vi "drawVessel.vi"(2 "alpha":dbl[](array[numeric]), 3 "u":dbl[](array[numeric])) -> (1 "?":picture)   [LabVIEW 2014]
uses:
  <vilib>/imath/engines/lvmath2/RunTimeEngine/NodeEndStatement/NIMS_NodeEndStatement_Output.vi
  <instcachedir>/0/NIMS_NodeEndStatement_Output_53EC0D466D134D7ABD903AC30B43404B.lvgen/NIMS_NodeEndStatement_Output_53EC0D466D134D7ABD903AC30B43404B_001.vi
  <vilib>/imath/engines/lvmath2/RunTimeEngine/ErrorHandling/NIMS_Finalize Error.vi
panel:
  out "?":picture
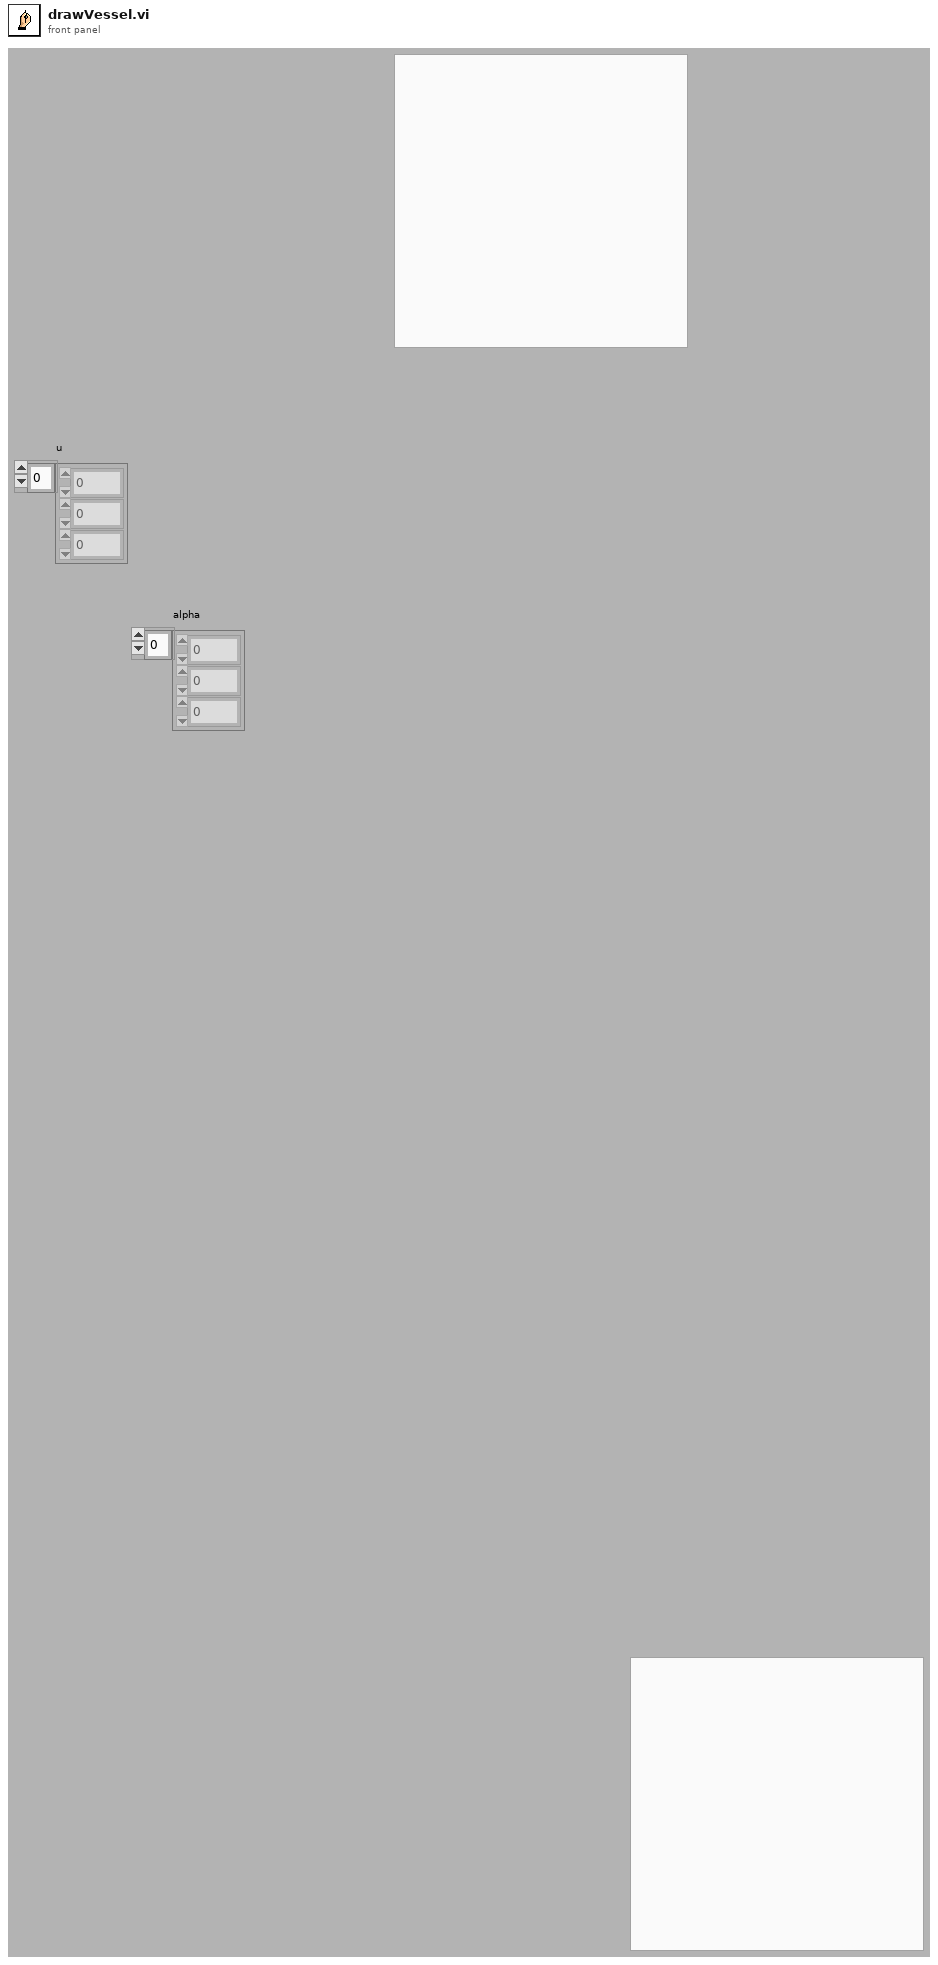
[diagram p1: front panel]
types:
  T1 = cluster{"Width":u16, "Style":enum32{"Solid", "Dash", "Dot", "DashDot", "DashDotDot"}}
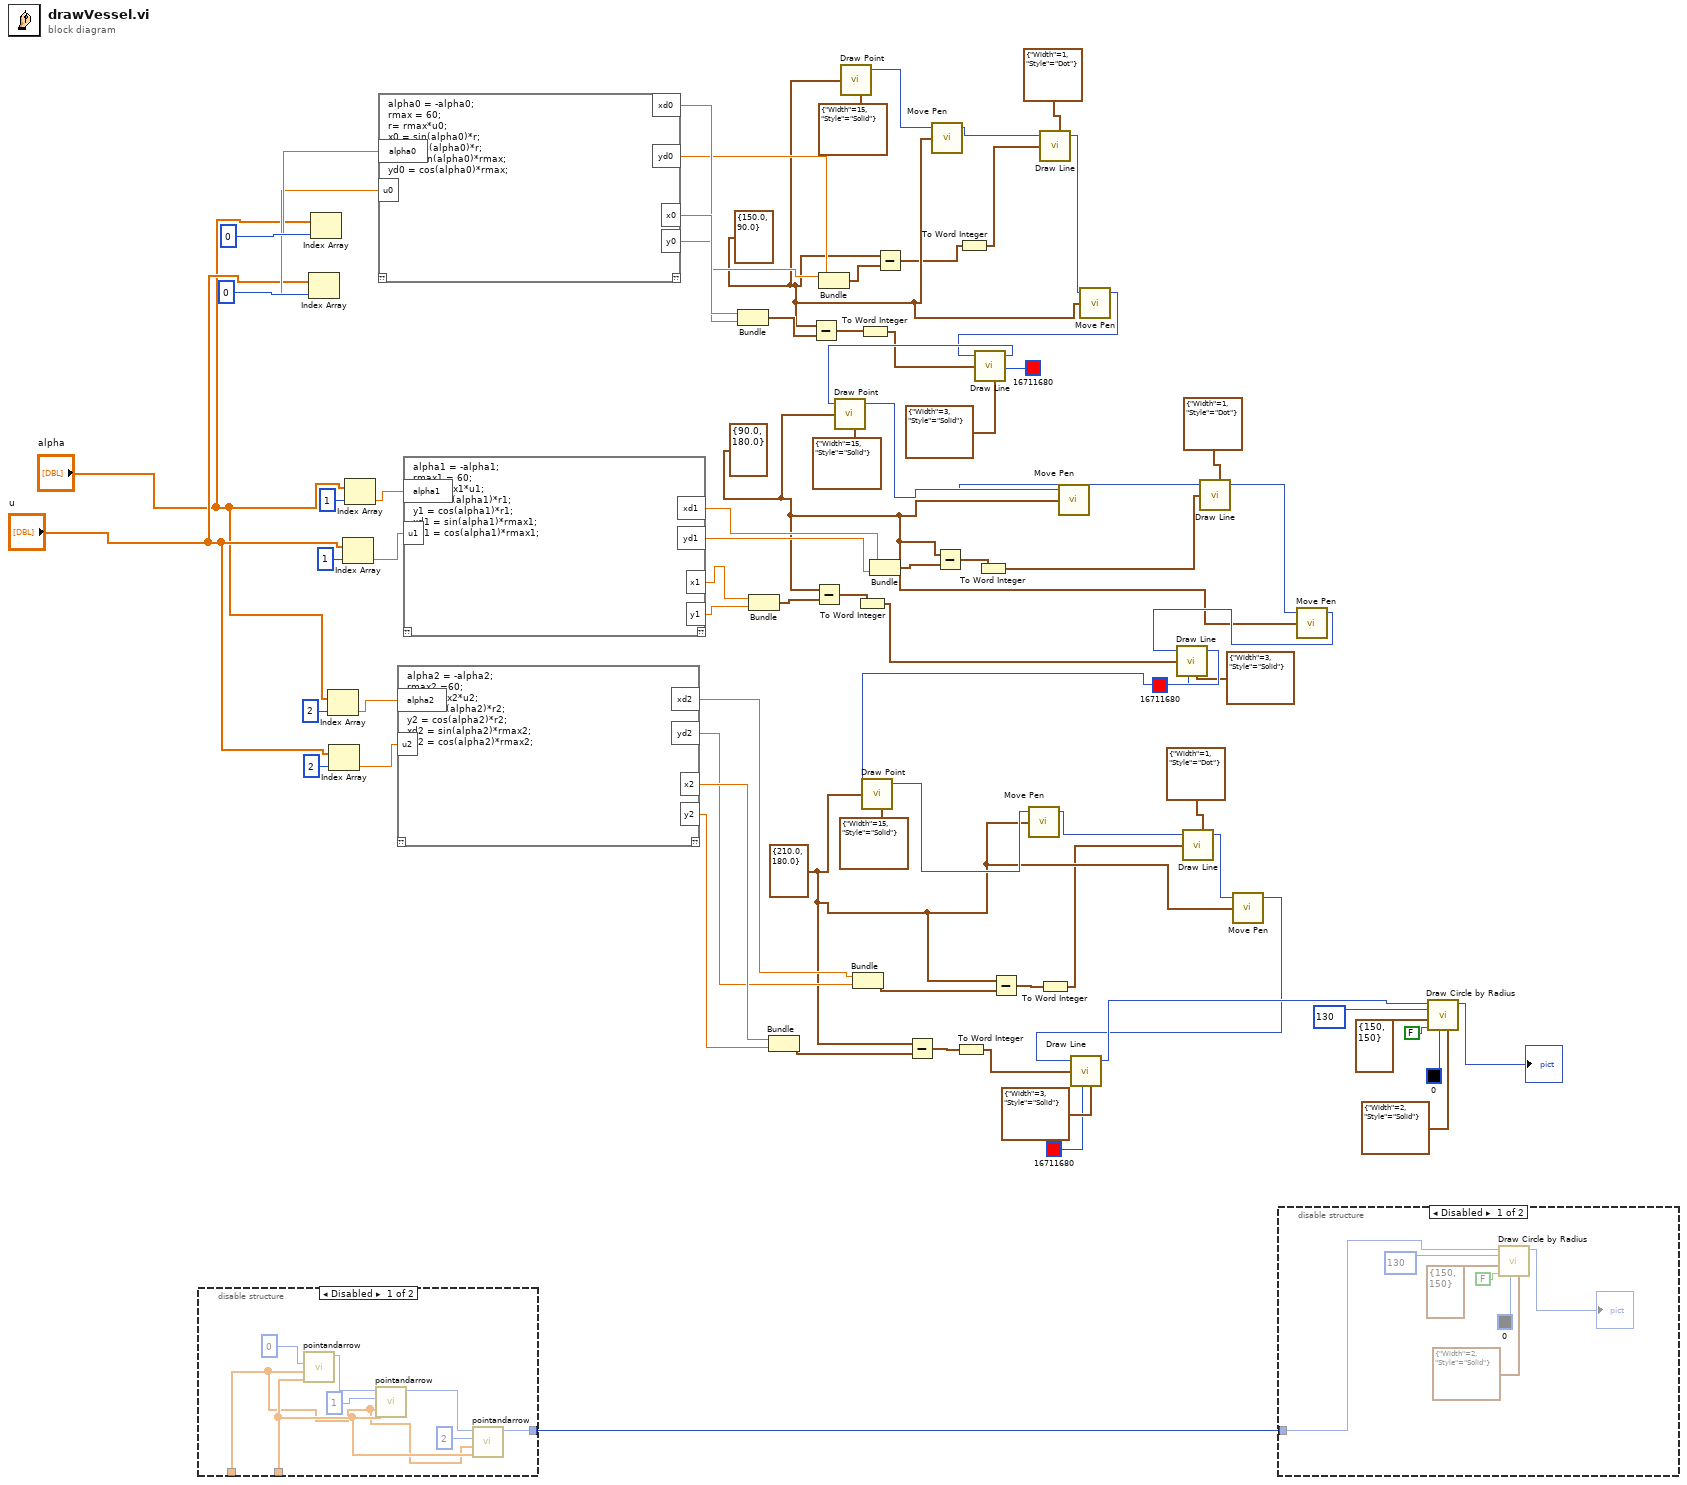
[diagram p0: block diagram]
diagram:
  w31 = cluster{dbl, dbl} {150.0, 90.0} ("new position")
  w18 = cluster{dbl, dbl} {210.0, 180.0} ("new position")
  w23 = cluster{dbl, dbl} {90.0, 180.0} ("new position")
  n1 = disable-structure shown="Disabled" {
    disable-tunnel: [w85 _] -> w81
    disable-tunnel: _ -> [w84 _]
    disable-tunnel: _ -> [w83 _]
    frame Disabled {
      n2 = call "pointandarrow.vi"("alpha"=w84, "u"=w83, "index"=0) -> ("new picture"=w88:picture)  [unwired: 8 in]
      n3 = call "pointandarrow.vi"("alpha"=w84, "u"=w83, "index"=1, "picture"=w88) -> ("new picture"=w82:picture)  [unwired: 7 in]
      n4 = call "pointandarrow.vi"("alpha"=w84, "u"=w83, "index"=2, "picture"=w82) -> ("new picture"=w85:picture)  [unwired: 7 in]
    }
    frame Enabled {
    }
  }
  n5 = Index Array(array="u", index=0) -> (element=w7:dbl)
  n6 = Index Array(array="alpha", index=0) -> (element=w8:dbl)
  n7 = Index Array(array="alpha", index=2) -> (element=w4:dbl)
  n8 = Index Array(array="u", index=2) -> (element=w3:dbl)
  n9 = Index Array(array="u", index=1) -> (element=w5:dbl)
  n10 = Index Array(array="alpha", index=1) -> (element=w6:dbl)
  n11 = mathscript code="alpha0 = -alpha0;\nrmax = 60;\nr= rmax*u0;\nx0 = sin(alpha0)*r;\ny0 = cos(alpha0)*r;\nxd0 = sin(alpha0)*rmax;\nyd0 = cos(alpha0)*rmax;"("alpha0"=w8, "u0"=w7) -> ("x0"=w63:dbl, "y0"=w62:dbl, "xd0"=w33:dbl, "yd0"=w32:dbl)  [unwired: 1 in, 1 out]
  n12 = mathscript code="alpha2 = -alpha2;\nrmax2 =60;\nr2= rmax2*u2;\nx2 = sin(alpha2)*r2;\ny2 = cos(alpha2)*r2;\nxd2 = sin(alpha2)*rmax2;\nyd2 = cos(alpha2)*rmax2;"("alpha2"=w4, "u2"=w3) -> ("x2"=w69:dbl, "y2"=w68:dbl, "xd2"=w19:dbl, "yd2"=w20:dbl)  [unwired: 1 in, 1 out]
  n13 = mathscript code="alpha1 = -alpha1;\nrmax1 = 60;\nr1= rmax1*u1;\nx1 = sin(alpha1)*r1;\ny1 = cos(alpha1)*r1;\nxd1 = sin(alpha1)*rmax1;\nyd1 = cos(alpha1)*rmax1;"("alpha1"=w6, "u1"=w5) -> ("x1"=w71:dbl, "y1"=w72:dbl, "xd1"=w26:dbl, "yd1"=w25:dbl)  [unwired: 1 in, 1 out]
  n14 = Bundle("x0"=w63, "y0"=w62) -> (w64:cluster{"x0":dbl, "y0":dbl})  [unwired: 1 in]
  n15 = Bundle("x1"=w71, "y1"=w72) -> (w70:cluster{"x1":dbl, "y1":dbl})  [unwired: 1 in]
  n16 = Bundle("x2"=w69, "y2"=w68) -> (w73:cluster{"x2":dbl, "y2":dbl})  [unwired: 1 in]
  n17 = Subtract(x=w31, y=w64) -> (x-y=w65:cluster{dbl, dbl})
  n18 = Subtract(x=w23, y=w70) -> (x-y=w75:cluster{dbl, dbl})
  n19 = Bundle("xd0"=w33, "yd0"=w32) -> (w34:cluster{"xd0":dbl, "yd0":dbl})  [unwired: 1 in]
  n20 = call <vilib>:"Draw Point.vi"("point(x,y)"=w31, "pen"=T1 {"Width"=15, "Style"=enum."Solid"}) -> ("new picture"=w60:picture)  [unwired: 7 in]
  n21 = Bundle("xd2"=w19, "yd2"=w20) -> (w21:cluster{"xd2":dbl, "yd2":dbl})  [unwired: 1 in]
  n22 = To Word Integer(number=w75) -> (16bit integer=w44:cluster{i16, i16})
  n23 = To Word Integer(number=w65) -> (16bit integer=w51:cluster{i16, i16})
  n24 = Bundle("xd1"=w26, "yd1"=w25) -> (w27:cluster{"xd1":dbl, "yd1":dbl})  [unwired: 1 in]
  n25 = Subtract(x=w31, y=w34) -> (x-y=w30:cluster{dbl, dbl})
  n26 = Subtract(x=w18, y=w73) -> (x-y=w74:cluster{dbl, dbl})
  n27 = call <vilib>:"Move Pen.vi"("new position"=w31, "picture"=w60) -> ("new picture"=w52:picture)  [unwired: 3 in]
  n28 = Subtract(x=w23, y=w27) -> (x-y=w28:cluster{dbl, dbl})
  n29 = To Word Integer(number=w74) -> (16bit integer=w37:cluster{i16, i16})
  n30 = To Word Integer(number=w30) -> (16bit integer=w29:cluster{i16, i16})
  n31 = To Word Integer(number=w28) -> (16bit integer=w24:cluster{i16, i16})
  n32 = Subtract(x=w18, y=w21) -> (x-y=w22:cluster{dbl, dbl})
  n33 = call <vilib>:"Draw Line.vi"("picture"=w52, "end point"=w29, "pen"=T1 {"Width"=1, "Style"=enum."Dot"}) -> ("new picture"=w49:picture)  [unwired: 6 in]
  n34 = To Word Integer(number=w22) -> (16bit integer=w17:cluster{i16, i16})
  n35 = call <vilib>:"Move Pen.vi"("new position"=w31, "picture"=w49) -> ("new picture"=w48:picture)  [unwired: 3 in]
  n36 = call <vilib>:"Draw Line.vi"("picture"=w48, "end point"=w51, "color(black)"=u32 16711680, "pen"=T1 {"Width"=3, "Style"=enum."Solid"}) -> ("new picture"=w56:picture)  [unwired: 5 in]
  n37 = call <vilib>:"Draw Point.vi"("picture"=w56, "point(x,y)"=w23, "pen"=T1 {"Width"=15, "Style"=enum."Solid"}) -> ("new picture"=w57:picture)  [unwired: 6 in]
  n38 = call <vilib>:"Move Pen.vi"("new position"=w23, "picture"=w57) -> ("new picture"=w45:picture)  [unwired: 3 in]
  n39 = call <vilib>:"Draw Line.vi"("picture"=w45, "end point"=w24, "pen"=T1 {"Width"=1, "Style"=enum."Dot"}) -> ("new picture"=w46:picture)  [unwired: 6 in]
  n40 = disable-structure shown="Disabled" {
    disable-tunnel: w81 -> [w90 _]
    frame Disabled {
      n41 = call <vilib>:"Draw Circle by Radius.vi"("pen"=T1 {"Width"=2, "Style"=enum."Solid"}, "color(black)"=u32 0, "fill?(F)"=FALSE, "pixel center"=cluster{"horizontal":i16, "vertical":i16} {"horizontal"=150, "vertical"=150}, "radius"=i16 130, "picture"=w90) -> ("new picture"=→"?":picture)  [unwired: 5 in]
    }
    frame Enabled {
    }
  }
  n42 = call <vilib>:"Move Pen.vi"("new position"=w23, "picture"=w46) -> ("new picture"=w43:picture)  [unwired: 3 in]
  n43 = call <vilib>:"Draw Line.vi"("picture"=w43, "end point"=w44, "color(black)"=u32 16711680, "pen"=T1 {"Width"=3, "Style"=enum."Solid"}) -> ("new picture"=w42:picture)  [unwired: 5 in]
  n44 = call <vilib>:"Draw Point.vi"("picture"=w42, "point(x,y)"=w18, "pen"=T1 {"Width"=15, "Style"=enum."Solid"}) -> ("new picture"=w55:picture)  [unwired: 6 in]
  n45 = call <vilib>:"Move Pen.vi"("new position"=w18, "picture"=w55) -> ("new picture"=w36:picture)  [unwired: 3 in]
  n46 = call <vilib>:"Draw Line.vi"("picture"=w36, "end point"=w17, "pen"=T1 {"Width"=1, "Style"=enum."Dot"}) -> ("new picture"=w38:picture)  [unwired: 6 in]
  n47 = call <vilib>:"Move Pen.vi"("new position"=w18, "picture"=w38) -> ("new picture"=w35:picture)  [unwired: 3 in]
  n48 = call <vilib>:"Draw Line.vi"("picture"=w35, "end point"=w37, "color(black)"=u32 16711680, "pen"=T1 {"Width"=3, "Style"=enum."Solid"}) -> ("new picture"=w66:picture)  [unwired: 5 in]
  n49 = call <vilib>:"Draw Circle by Radius.vi"("pen"=T1 {"Width"=2, "Style"=enum."Solid"}, "color(black)"=u32 0, "fill?(F)"=FALSE, "pixel center"=cluster{"horizontal":i16, "vertical":i16} {"horizontal"=150, "vertical"=150}, "radius"=i16 130, "picture"=w66) -> ("new picture"=→"?":picture)  [unwired: 5 in]
